vi "SwitchedCameraData.vi"() -> ()   [LabVIEW 2017]
panel:
  in  "SwitchedCameraName":string
  in  "ActiveSwitchedCamera":string
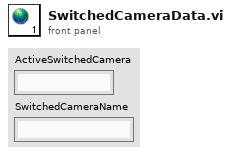
[diagram p1: front panel]
diagram:
